vi "Example - String to Scaled Value Utility.vi"() -> ()   [LabVIEW 2013, in "Mercury iXX.lvlib"]
uses:
  Program Files (x86)/National Instruments/LabVIEW 2017/instr.lib/Mercury iXX/Mercury iXX.lvlib
  Program Files (x86)/National Instruments/LabVIEW 2017/instr.lib/Mercury iXX/Public/Libraries/System/Open/Open Device.vi
  Program Files (x86)/National Instruments/LabVIEW 2017/instr.lib/Mercury iXX/Public/Libraries/System.lvlib
  Program Files (x86)/National Instruments/LabVIEW 2017/instr.lib/Mercury iXX/Public/Libraries/System/Open/Open System.vi
  Program Files (x86)/National Instruments/LabVIEW 2017/instr.lib/Mercury iXX/Public/Libraries/System/Read/Time (Read).vi
  Program Files (x86)/National Instruments/LabVIEW 2017/instr.lib/Mercury iXX/Public/Libraries/System/Read/DateTime (Read).vi
  Program Files (x86)/National Instruments/LabVIEW 2017/instr.lib/Mercury iXX/Public/Controls/Comms Transport Layer.ctl
  Program Files (x86)/National Instruments/LabVIEW 2017/instr.lib/Mercury iXX/Public/Libraries/System/Read/Date (Read).vi
  Program Files (x86)/National Instruments/LabVIEW 2017/instr.lib/Mercury iXX/Public/Libraries/System/Read/Flash Space (Read).vi
  Program Files (x86)/National Instruments/LabVIEW 2017/instr.lib/Mercury iXX/Public/Libraries/System/Read/Catalogue (Read).vi
  Program Files (x86)/National Instruments/LabVIEW 2017/instr.lib/Mercury iXX/Public/Controls/ISOBus Address.ctl
  Program Files (x86)/National Instruments/LabVIEW 2017/instr.lib/Mercury iXX/Public/Libraries/Heater/Configuration/Read/Heater Device (Read).vi
  Program Files (x86)/National Instruments/LabVIEW 2017/instr.lib/Mercury iXX/Public/Libraries/Heater.lvlib
  Program Files (x86)/National Instruments/LabVIEW 2017/instr.lib/Mercury iXX/Public/Libraries/Heater/Configuration/Read/Serial Number (Read).vi
  Program Files (x86)/National Instruments/LabVIEW 2017/instr.lib/Mercury iXX/Public/Libraries/Heater/Configuration/Read/Voltage Limit (Read).vi
  Program Files (x86)/National Instruments/LabVIEW 2017/instr.lib/Mercury iXX/Public/Libraries/Heater/Configuration/Read/Nominal Resistance (Read).vi
  Program Files (x86)/National Instruments/LabVIEW 2017/instr.lib/Mercury iXX/Public/Libraries/Heater/Configuration/Read/Maximum Power (Read).vi
  Program Files (x86)/National Instruments/LabVIEW 2017/instr.lib/Mercury iXX/Public/Libraries/Heater/Signals/Read/Voltage (Read).vi
  Program Files (x86)/National Instruments/LabVIEW 2017/instr.lib/Mercury iXX/Public/Libraries/Heater/Signals/Read/Power (Read).vi
  Program Files (x86)/National Instruments/LabVIEW 2017/instr.lib/Mercury iXX/Public/Libraries/Heater/Signals/Read/Current (Read).vi
  Program Files (x86)/National Instruments/LabVIEW 2017/instr.lib/Mercury iXX/Public/Libraries/Heater/Configuration/Read/Nickname (Read).vi
  Program Files (x86)/National Instruments/LabVIEW 2017/instr.lib/Mercury iXX/Public/Libraries/System/Read/HVer (Read).vi
  Program Files (x86)/National Instruments/LabVIEW 2017/instr.lib/Mercury iXX/Public/Libraries/System/Read/FVer (Read).vi
  Program Files (x86)/National Instruments/LabVIEW 2017/instr.lib/Mercury iXX/Public/Libraries/System/Read/Serial Number (Read).vi
  Program Files (x86)/National Instruments/LabVIEW 2017/instr.lib/Mercury iXX/Public/Controls/SI Prefix.ctl
  Program Files (x86)/National Instruments/LabVIEW 2017/instr.lib/Mercury iXX/Public/Controls/Manufacturing Data.ctl
  Program Files (x86)/National Instruments/LabVIEW 2017/instr.lib/Mercury iXX/Public/Controls/Unit String.ctl
  Program Files (x86)/National Instruments/LabVIEW 2017/instr.lib/Mercury iXX/Public/Libraries/Heater/Controls/Heater Signals Cluster.ctl
  Program Files (x86)/National Instruments/LabVIEW 2017/instr.lib/Mercury iXX/Public/Libraries/Heater/Controls/Heater Device (Read).ctl
panel:
  in  "Mercury Functions":enum32{"System", "Heater"}(tab)
  out "time stamp":timestamp
  out "Free Space":i32 caption="Free Space (KB)"
  out "String":string="NORM" caption="User Mode"
  out "Date":string
  out "Time":string
  out "Hardware Version":string
  out "Firmware Version":string
  out "Serial Number":string
  out "Devices":string[](array[string])
  out "S/W Version(s)":string[](array[string])
  out "Serial Number(s)":string[](array[string])
  out "# of Instruments":i32
  out "Heater Device Settings":T1
  out "Htr C Unit":T4
  out "Htr P Unit":T4
  out "Htr V Unit":T4
  out "Htr Current":dbl
  out "Htr Power":dbl
  out "Htr Voltage":dbl
  out "Power Unit":T4
  out "Volt Unit":T4
  out "Res Unit":T4
  out "Maximum Power":dbl
  out "Htr Resistance":dbl
  out "Htr Voltage Limit":dbl
  out "Htr S/N":string
  out "Htr Nickname":string
  out "Value":dbl format="%#.6f"
  out "Unit (with prefix)":T4
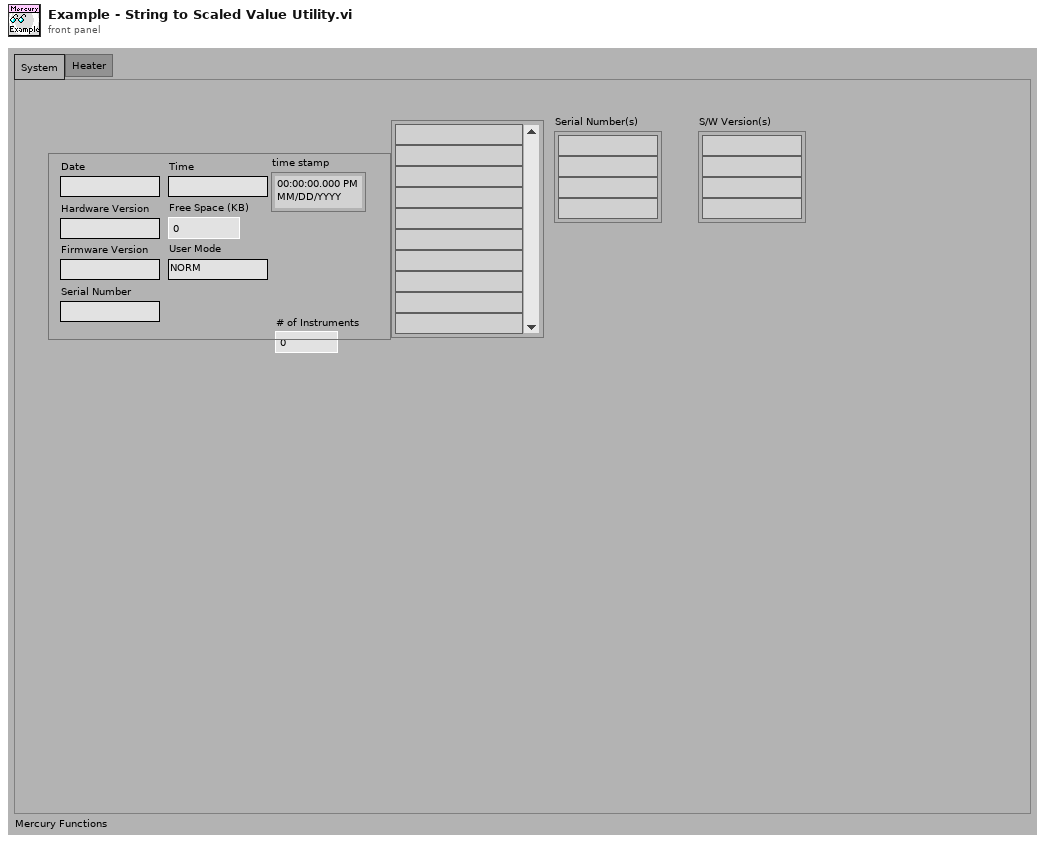
[diagram p1: front panel]
types:
  T1 = typedef "Mercury iXX.lvlib/Heater.lvlib/Heater Device (Read).ctl" = cluster{"Manufacturing":T2, "Nickname":string, "Voltage Limit":string, "Nominal Resistance":string, "Maximum Power":string, "Heater Signals":T3, "Status":string}
  T2 = typedef "Mercury iXX.lvlib/Manufacturing Data.ctl" = cluster{"Hardware Version":string, "Firmware Version":string, "Serial Number":string}
  T3 = typedef "Mercury iXX.lvlib/Heater.lvlib/Heater Signals Cluster.ctl" = cluster{"Voltage":string, "Current":string, "Power":string}
  T4 = typedef "Mercury iXX.lvlib/Unit String.ctl" = string
  T5 = typedef "Mercury iXX.lvlib/SI Prefix.ctl" = enum16{"n", "µ", "m", "No Prefix", "k", "M", "G"}
  T6 = typedef "Mercury iXX.lvlib/ISOBus Address.ctl" = i32
  T7 = typedef "Mercury iXX.lvlib/Comms Transport Layer.ctl" = enum16{"Ethernet TCP/IP", "USB", "ISOBus - RS-232", "GPIB"}
  T8 = typedef "Mercury iXX.lvlib/Mercury Reference.ctl" = cluster{"Comms":refnum<visa-resource-name>, "Device ID":string[], "Comms Layer":T7, "Command":string, "Query reference":T9}
  T9 = typedef "Mercury iXX.lvlib/Query Dynamic Reference.ctl" = refnum<vi>
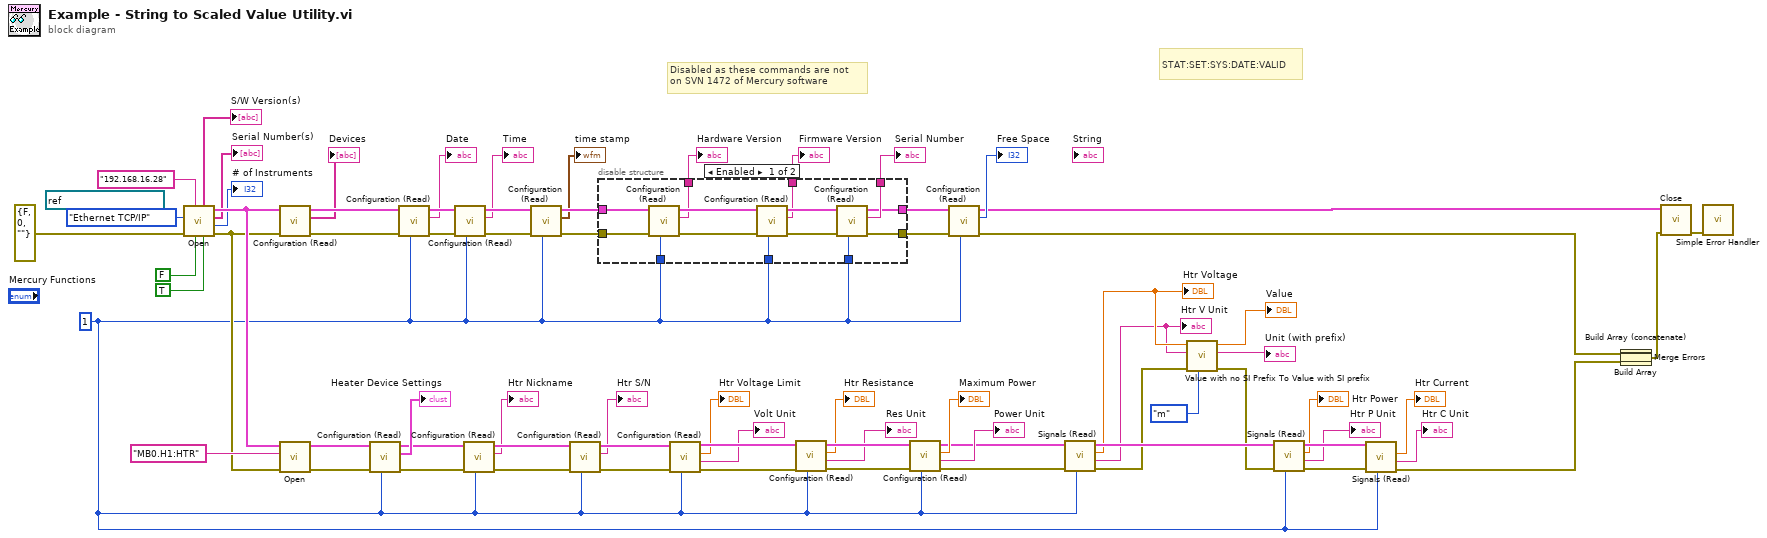
[diagram p0: block diagram]
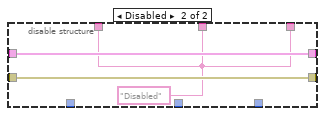
[diagram p2: hidden frame]
diagram:
  w12 = T6 1 ("ISOBUS address")
  (unwired) refnum<visa-resource-name> "COM1" ("VISA resource name")
  # "Disabled as these commands are not \non SVN 1472 of Mercury software"
  # "STAT:SET:SYS:DATE:VALID"
  n1 = call-poly "Open.vi"("Clear Previous Connections (False)"=TRUE ("Clear Previous Connections (True)"), "ID Query (True)"=FALSE, "IP Address"="192.168.16.28", "error in (no error)"=errorcluster {"status"=FALSE, "code"=0, "source"=""}, "Comms Layer"=Comms_Transport_Layer."Ethernet TCP/IP") -> ("error out"=w13:errorcluster, "# of Instruments"=→"# of Instruments":i32, "Serial Number(s)"=→"Serial Number(s)":string[], "Mercury Reference Out"=w23:T8, "S/W Version(s)"=→"S/W Version(s)":string[])  [unwired: 2 in]
  n2 = call-poly "Configuration (Read).vi"("error in"=w13, "Mercury Reference In"=w23) -> ("error out"=w35:errorcluster, "Devices"=→"Devices":string[], "Mercury Reference Out"=w36:T8)  [unwired: 1 in, 6 out]
  n3 = call-poly "Open.vi"("error in (no error)"=w13, "Device Identifier"="MB0.H1:HTR", "Mercury Reference In"=w23) -> ("error out"=w59:errorcluster, "Mercury Reference Out"=w60:T8)  [unwired: 1 in, 6 out]
  n4 = call-poly "Configuration (Read).vi"("ISOBUS address"=w12, "error in"=w59, "Mercury Reference In"=w60) -> ("error out"=w32:errorcluster, "Device Details"=→"Heater Device Settings":T1, "Mercury Reference Out"=w33:T8)  [unwired: 6 out]
  n5 = call-poly "Configuration (Read).vi"("ISOBUS address"=w12, "error in"=w35, "Mercury Reference In"=w36) -> ("error out"=w73:errorcluster, "Date"=→"Date":string, "Mercury Reference Out"=w74:T8)  [unwired: 6 out]
  n6 = call-poly "Configuration (Read).vi"("ISOBUS address"=w12, "error in"=w73, "Mercury Reference In"=w74) -> ("error out"=w71:errorcluster, "Time"=→"Time":string, "Mercury Reference Out"=w72:T8)  [unwired: 6 out]
  n7 = call-poly "Configuration (Read).vi"("ISOBUS address"=w12, "error in"=w32, "Mercury Reference In"=w33) -> ("error out"=w30:errorcluster, "Nickname"=→"Htr Nickname":string, "Mercury Reference Out"=w31:T8)  [unwired: 6 out]
  n8 = call-poly "Configuration (Read).vi"("ISOBUS address"=w12, "error in"=w71, "Mercury Reference In"=w72) -> ("error out"=w69:errorcluster, "time stamp"=→"time stamp":timestamp, "Mercury Reference Out"=w70:T8)  [unwired: 6 out]
  n9 = call-poly "Configuration (Read).vi"("ISOBUS address"=w12, "error in"=w30, "Mercury Reference In"=w31) -> ("error out"=w57:errorcluster, "Serial Number"=→"Htr S/N":string, "Mercury Reference Out"=w58:T8)  [unwired: 6 out]
  n10 = disable-structure shown="Enabled" {
    disable-tunnel: w70 -> [w86 w91]
    disable-tunnel: w69 -> [w85 w90]
    disable-tunnel: [w75 w89] -> w26
    disable-tunnel: [w82 w89] -> w25
    disable-tunnel: [w81 w89] -> w24
    disable-tunnel: [w80 w91] -> w68
    disable-tunnel: [w79 w90] -> w67
    disable-tunnel: w12 -> [w78 _]
    disable-tunnel: w12 -> [w77 _]
    disable-tunnel: w12 -> [w76 _]
    frame Enabled {
      n11 = call-poly "Configuration (Read).vi"("ISOBUS address"=w78, "error in"=w85, "Mercury Reference In"=w86) -> ("error out"=w83:errorcluster, "Hardware Version"=w75:string, "Mercury Reference Out"=w84:T8)  [unwired: 6 out]
      n12 = call-poly "Configuration (Read).vi"("ISOBUS address"=w77, "error in"=w83, "Mercury Reference In"=w84) -> ("error out"=w87:errorcluster, "Firmware Version"=w82:string, "Mercury Reference Out"=w88:T8)  [unwired: 6 out]
      n13 = call-poly "Configuration (Read).vi"("ISOBUS address"=w76, "error in"=w87, "Mercury Reference In"=w88) -> ("error out"=w79:errorcluster, "Serial Number"=w81:string, "Mercury Reference Out"=w80:T8)  [unwired: 6 out]
    }
    frame Disabled {
      w89 = "Disabled" ("Firmware Version")
    }
  }
  "Hardware Version" <- w26
  "Firmware Version" <- w25
  "Serial Number" <- w24
  n14 = call-poly "Configuration (Read).vi"("ISOBUS address"=w12, "error in"=w57, "Mercury Reference In"=w58) -> ("error out"=w56:errorcluster, "Unit"=→"Volt Unit":T4, "Voltage Limit"=→"Htr Voltage Limit":dbl, "Mercury Reference Out"=w53:T8)  [unwired: 5 out]
  n15 = call-poly "Configuration (Read).vi"("ISOBUS address"=w12, "error in"=w56, "Mercury Reference In"=w53) -> ("error out"=w55:errorcluster, "Unit"=→"Res Unit":T4, "Nominal Resistance"=→"Htr Resistance":dbl, "Mercury Reference Out"=w54:T8)  [unwired: 5 out]
  n16 = call-poly "Configuration (Read).vi"("ISOBUS address"=w12, "error in"=w55, "Mercury Reference In"=w54) -> ("error out"=w45:errorcluster, "Unit"=→"Power Unit":T4, "Maximum Power"=→"Maximum Power":dbl, "Mercury Reference Out"=w46:T8)  [unwired: 5 out]
  n17 = call-poly "Configuration (Read).vi"("ISOBUS address"=w12, "error in"=w67, "Mercury Reference In"=w68) -> ("error out"=w10:errorcluster, "Free Space"=→"Free Space":i32, "Mercury Reference Out"=w11:T8)  [unwired: 6 out]
  n18 = call-poly "Signals (Read).vi"("ISOBUS address"=w12, "error in"=w45, "Mercury Reference In"=w46) -> ("error out"=w8:errorcluster, "Unit"=w5:T4, "Voltage"=w6:dbl, "Mercury Reference Out"=w44:T8)  [unwired: 5 out]
  "Htr Voltage" <- w6
  "Htr V Unit" <- w5
  n19 = call "Value with no SI Prefix To Value with SI prefix.vi"("Output Prefix"=SI_Prefix."m", "error in"=w8, "Unit In"=w5, "Scaled Value"=w6) -> ("error out"=w7:errorcluster, "Unit (with prefix)"=→"Unit (with prefix)":T4, "Value"=→"Value":dbl)  [unwired: 5 out]
  n20 = call-poly "Signals (Read).vi"("ISOBUS address"=w12, "error in"=w7, "Mercury Reference In"=w44) -> ("error out"=w42:errorcluster, "Unit"=→"Htr P Unit":T4, "Power"=→"Htr Power":dbl, "Mercury Reference Out"=w43:T8)  [unwired: 5 out]
  n21 = call-poly "Signals (Read).vi"("ISOBUS address"=w12, "error in"=w42, "Mercury Reference In"=w43) -> ("error out"=w9:errorcluster, "Unit"=→"Htr C Unit":T4, "Current"=→"Htr Current":dbl)  [unwired: 6 out]
  n22 = Build Array(w10, w9) -> (w14:errorcluster[])
  n23 = Build Array (concatenate)(w14) -> (w1:errorcluster[])
  n24 = Merge Errors(w1) -> (w61:errorcluster)
  n25 = call "Close.vi"("error in (no error)"=w61, "Mercury Reference"=w11) -> ("error out"=w17:errorcluster)  [unwired: 9 out]
  n26 = call <vilib>:"Simple Error Handler.vi"("error in (no error)"=w17) -> ()  [unwired: 1 in, 8 out]
